vi "Read Fluke Configuration.vi"(8 "error in (no error)":errorcluster, 11 "Fluke 1586A Driver in":refnum<class "Fluke 1586A Driver.lvclass">) -> (0 "error out":errorcluster, 2 "Configuration":T1={"Channels"="201:203"}, 3 "Fluke 1586A Driver out":refnum<class "Fluke 1586A Driver.lvclass">)   [LabVIEW 2019, in "Fluke 1586A Driver.lvclass"]
uses:
  Fluke 1586A Driver.lvclass
  C:/GitHub/NHMFL_Core/Libraries/Instruments/Instrument Driver/Instrument Driver.lvclass
  Fluke Configuration.ctl
  Instrument Driver/Read User configuration.vi
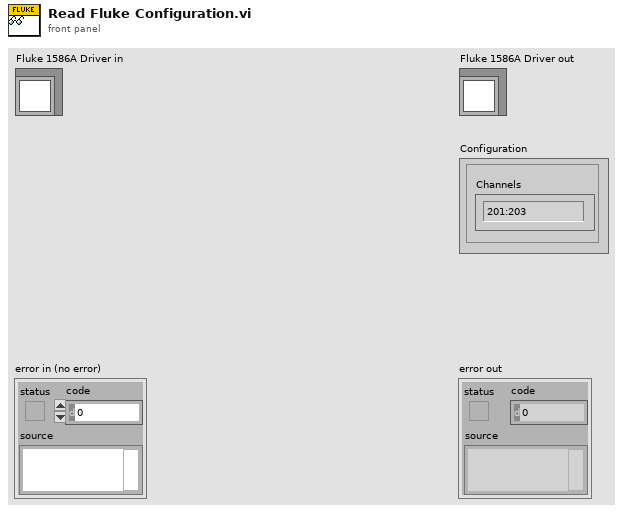
[diagram p1: front panel]
types:
  T1 = typedef "Fluke Configuration.ctl" = cluster{"Channels":string}
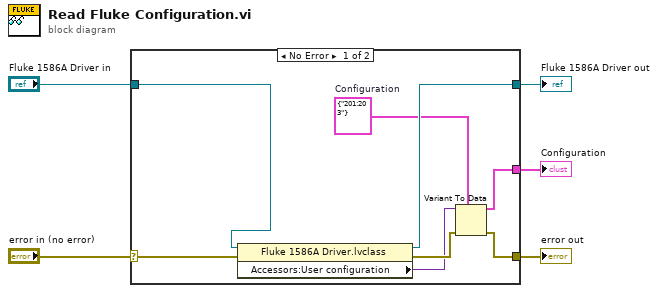
[diagram p0: block diagram]
diagram:
  n1 = case shown="No Error" "error in (no error)" {
    selector: "error in (no error)" -> [w13 w14]
    tunnel: [w9 w14] -> w4
    tunnel: [w11 w15] -> w2
    tunnel: "Fluke 1586A Driver in" -> [w12 w15]
    tunnel: [w6 _] -> w1
    frame No Error {
      w7 = T1 {"Channels"="201:203"}  # Configuration
      n2 = property class="Fluke 1586A Driver.lvclass"(reference=w12, error in=w13) -> (reference out=w11:refnum<class "Fluke 1586A Driver.lvclass">, error out=w10:errorcluster, "Accessors:User configuration"=w8:variant)
      n3 = Variant To Data(error in=w10, type=w7, Variant=w8) -> (data=w6:T1, error out=w9:errorcluster)
    }
    frame Error {
    }
  }
  "error out" <- w4
  "Fluke 1586A Driver out" <- w2
  "Configuration" <- w1
